vi "Revision Query Core.vi"(8 "error in (no error)":errorcluster, 11 "IVI_DMM-3458A in":refnum<class "IVI_DMM-3458A.lvclass">) -> (0 "error out":errorcluster, 1 "Firmware Revision":string, 2 "Driver Revision":string, 3 "IVI_DMM-3458A out":refnum<class "IVI_DMM-3458A.lvclass">)   [LabVIEW 2015, in "IVI_DMM.lvlib" / "IVI_DMM-3458A.lvclass"]
uses:
  IVI_DMM-3458A.lvclass
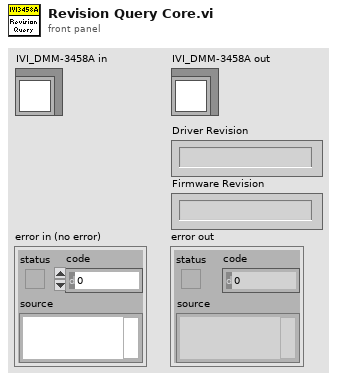
[diagram p1: front panel]
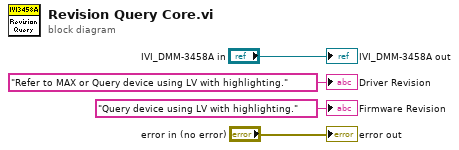
[diagram p0: block diagram]
diagram:
  "error out" <- "error in (no error)"
  "IVI_DMM-3458A out" <- "IVI_DMM-3458A in"
  "Driver Revision" <- "Refer to MAX or Query device using LV with highlighting." ("Driver Revision")
  "Firmware Revision" <- "Query device using LV with highlighting." ("Firmware Revision")
